vi "SPI Flash Erase Chip.vi"(9 "TimeOutMs":i32, 10 "SPIIndex":i32, 11 "DevHandle":i32) -> (3 "function return":i32)   [LabVIEW 2010, in "usb2spi.lvlib"]
doc: "int WINAPI SPI_FlashEraseChip(int DevHandle,int SPIIndex,int TimeOutMs);"
uses:
  usb2spi.lvlib
  USB2XXX/trunk/USB2XXX/USB2XXX/vs2019/Release/USB2XXX.dll
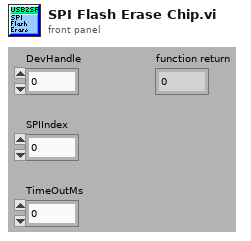
[diagram p1: front panel]
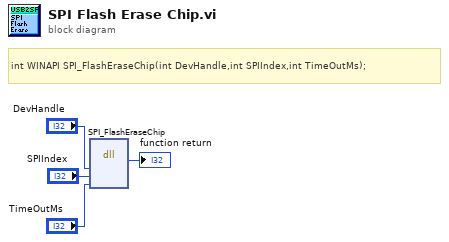
[diagram p0: block diagram]
diagram:
  # "int WINAPI SPI_FlashEraseChip(int DevHandle,int SPIIndex,int TimeOutMs);"
  n1 = dll-call lib="E:/Projects/USB2XXX/trunk/USB2XXX/USB2XXX/vs2019/Release/USB2XXX.*" fn="SPI_FlashEraseChip"("DevHandle"="DevHandle", "SPIIndex"="SPIIndex", "TimeOutMs"="TimeOutMs") -> (→"function return":i32)  [unwired: 6 in, 2 out]
